vi "ProdaNG.CreateProduct.vi"(8 "error in (no error)":errorcluster, 9 "serialNumber":string, 10 "ID":T2, 11 "dbHandle":i32) -> (0 "error out":errorcluster, 1 "Product out":T1, 3 "dbHandle out":i32)   [LabVIEW 2016]
doc: "This function returns a product structure for a product, which is identified by a part and a serial number.\nImportant information: The field 'individual' was taken over from the field 'allgemein' of the legacy data directly. Because of this most products have the value 0 further on and only a few the value 1. \nParameter:\nhandle is an Integer, which is returned by the function Login() at the creation of a new connection.\nwabcoPartId is the Id of the part.\nserialNumber is the serial number of the product for the part above.\nproduct is a pointer on a product structure, which is filled if the returncode is 0. The structure must be defined in the calling program.\n\nReturncodes:\n0 No error\n< 0 ORACLE Error code\n6 (ERROR_INVALID_HANDLE) in case of an invalid handle\n1403 Record does not exist"
uses:
  Controls/ProdaNG.Identification.ctl
  Controls/ProdaNG.Product.ctl
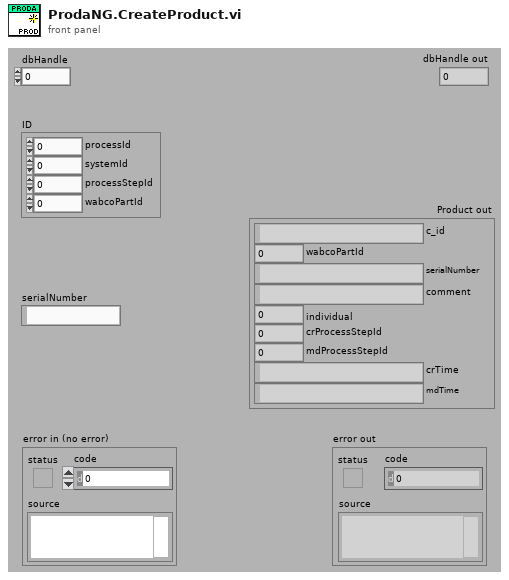
[diagram p1: front panel]
types:
  T1 = typedef "ProdaNG.Product.ctl" = cluster{"c_id":string, "wabcoPartId":i32, "serialNumber":string, "comment":string, "individual":i32, "crProcessStepId":i32, "mdProcessStepId":i32, "crTime":string, "mdTime":string}
  T2 = typedef "ProdaNG.Identification.ctl" = cluster{"processId":i32, "systemId":i32, "processStepId":i32, "wabcoPartId":i32}
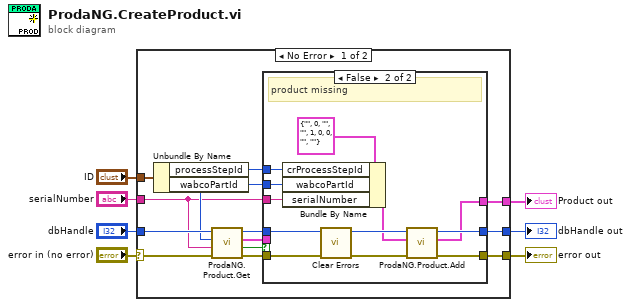
[diagram p0: block diagram]
diagram:
  n1 = case shown="No Error" "error in (no error)" {
    selector: "error in (no error)" -> [w20 w36]
    tunnel: [w17 w36] -> w6
    tunnel: "dbHandle" -> [w13 w35]
    tunnel: [w14 w35] -> w4
    tunnel: "serialNumber" -> [w8 _]
    tunnel: "ID" -> [w12 _]
    tunnel: [w9 _] -> w1
    frame No Error {
      n2 = Unbundle By Name(w12) -> ("processStepId"=w10:i32, "wabcoPartId"=w11:i32)
      n3 = call "ProdaNG.Product.Get.vi"("error in (no error)"=w20, "serialNumber"=w8, "wabcoPartId"=w11, "dbHandle"=w13) -> ("error out"=w19:errorcluster, "found"=w18:bool, "Product"=w16:T1, "dbHandle out"=w15:i32)  [unwired: 4 in]
      n4 = case shown="False" w18 {
        tunnel: w19 -> [w21 w34]
        tunnel: [w21 w32] -> w17
        tunnel: w16 -> [w23 _]
        tunnel: w15 -> [w22 w33]
        tunnel: [w22 w29] -> w14
        tunnel: w11 -> [_ w31]
        tunnel: w8 -> [_ w30]
        tunnel: w10 -> [_ w28]
        tunnel: [w23 w27] -> w9
        frame True {
          # "product exists"
        }
        frame False {
          # "product missing"
          n5 = Bundle By Name(cluster=T1 {"c_id"="", "wabcoPartId"=0, "serialNumber"="", "comment"="", "individual"=1, "crProcessStepId"=0, "mdProcessStepId"=0, "crTime"="", "mdTime"=""} ("Product"), "crProcessStepId"=w28, "wabcoPartId"=w31, "serialNumber"=w30) -> (w24:T1)
          n6 = call <vilib>:"Clear Errors.vi"("error in (no error)"=w34) -> ("error out"=w26:errorcluster)  [unwired: 5 in, 1 out]
          n7 = call "ProdaNG.Product.Add.vi"("error in (no error)"=w26, "Product"=w24, "dbHandle"=w33) -> ("error out"=w32:errorcluster, "Product out"=w27:T1, "dbHandle"=w29:i32)  [unwired: 6 in]
        }
      }
    }
    frame Error {
    }
  }
  "error out" <- w6
  "dbHandle out" <- w4
  "Product out" <- w1
